vi "Dynamic_Control_Demo.vi"() -> ()   [LabVIEW 2012]
uses:
  <vilib>/Simulation/Scripting/Companion Diagram/SimConfigNode/SimParams.ctl
  <vilib>/Simulation/Scripting/Companion Diagram/SimConfigNode/_simSolvers.ctl
  <vilib>/Simulation/Implementation/Shared/SIMSCR Execution Mode.ctl
  <vilib>/Simulation/Param Hierarchy/Typedefs/SIMPH Param Control Actions.ctl
  <vilib>/Simulation/Implementation/Shared/NILVSim_ParamChanged.vi
  <vilib>/Simulation/DataSources/Implementation/NILVSim Step.llb/SIM Step (scalar).vi
  <vilib>/Simulation/SignalArithmetic/Implementation/NILVSim Gain.llb/SIM Gain (scalar).vi
  <vilib>/Simulation/Utility/Implementation/SIM Halt.vi
  <vilib>/Simulation/DiscreteLinear/Implementation/NILVSim Discrete State Space Buffered.llb/SIM Discrete State Space Distributor (SISO CD).vi
  <vilib>/Simulation/SignalArithmetic/Implementation/NILVSim Gain.llb/SIM Gain (dot product).vi
  <vilib>/Simulation/DiscreteLinear/Implementation/NILVSim Discrete State Space Buffered.llb/SIM Discrete State Space Collector (SISO CD).vi
  <vilib>/Simulation/SignalDisplay/Implementation/NILVSim Time Waveform.llb/SIM Time Waveform (scalar).vi
  <vilib>/Simulation/Implementation/Shared/NILVSim_Manager.vi
  <vilib>/Simulation/Implementation/Shared/NILVSim_FinalizeModel.vi
  <vilib>/Simulation/Implementation/Shared/SIM Unbundle Sim Info.vi
  <vilib>/Utility/error.llb/Clear Errors.vi
  <vilib>/Simulation/Implementation/Shared/NILVSim_GetModelError.vi
  <vilib>/Simulation/Implementation/Shared/SIM Bundle Sim Info.vi
  <vilib>/Simulation/Implementation/Shared/SIMSH Read Queue.vi
  <vilib>/Simulation/Implementation/Shared/NILVSim_Initialize.vi
  <vilib>/Simulation/Utility/Implementation/NILVSim Get Time and IsAcceptedStep.vi
  <vilib>/Simulation/Scripting/Companion Diagram/SimConfigNode/SimDog.xnode
  <vilib>/Simulation/Implementation/XNodeFramework/SimXNode/SimX.xnode
  <vilib>/addons/Control Design/_Model Construction/Model Typedefs.llb/CD General Elements.ctl
  <vilib>/addons/Control Design/_Model Construction/NI_LinSys_Model Typedefs.lvlib
  <vilib>/addons/Control Design/_Model Construction/Model Typedefs.llb/CD State Space Model (MIMO).ctl
  <vilib>/Simulation/DiscreteLinear/Implementation/NILVSim Discrete State Space Buffered.llb/SIM Discrete State Space Buffered (SISO CD).vi
  <vilib>/Simulation/Implementation/Shared/NI_SIM_Implementation.lvlib
panel:
  in  "Halt?":bool
  out "Waveform Plot":waveform(dbl)(graph)={"t0"=timestamp(19414.600000000002 s since 1904-01-01), "dt"=1.0, "Y"=[0.0]}
  out "state x(k+1)":dbl[](array[numeric])
  out "state x(k)":dbl[](array[numeric])
  out "Output y(k)":dbl
  in  "Error IN":dbl(slide) scale=-90.0..90.0
  out "Controllability Matrix":dbl[][](array[numeric])=[[0.0029424877498334255, 0.008616646869548867, 0.014016016852462686, 0.019193532183387766], [0.05829906495647488, 0.05527735475623796, 0.052797981566245, 0.05083784073300338], [0.000983525405599516, 0.0029123179012991098, 0.004844756877997715, 0.006861898357198368], [0.019540617662783182, 0.019171356382024756, 0.019611979984952656, 0.02086921364939449]] format="%.2f"
  out "Feedback Gain (K)":dbl[](array[numeric])=[-63312112.22140336, 6720868.965421855, 193328496.30508494, -20246021.6652911]
  out "Discrete Model Out":picture
  out "Waveform Chart":dbl(graph)
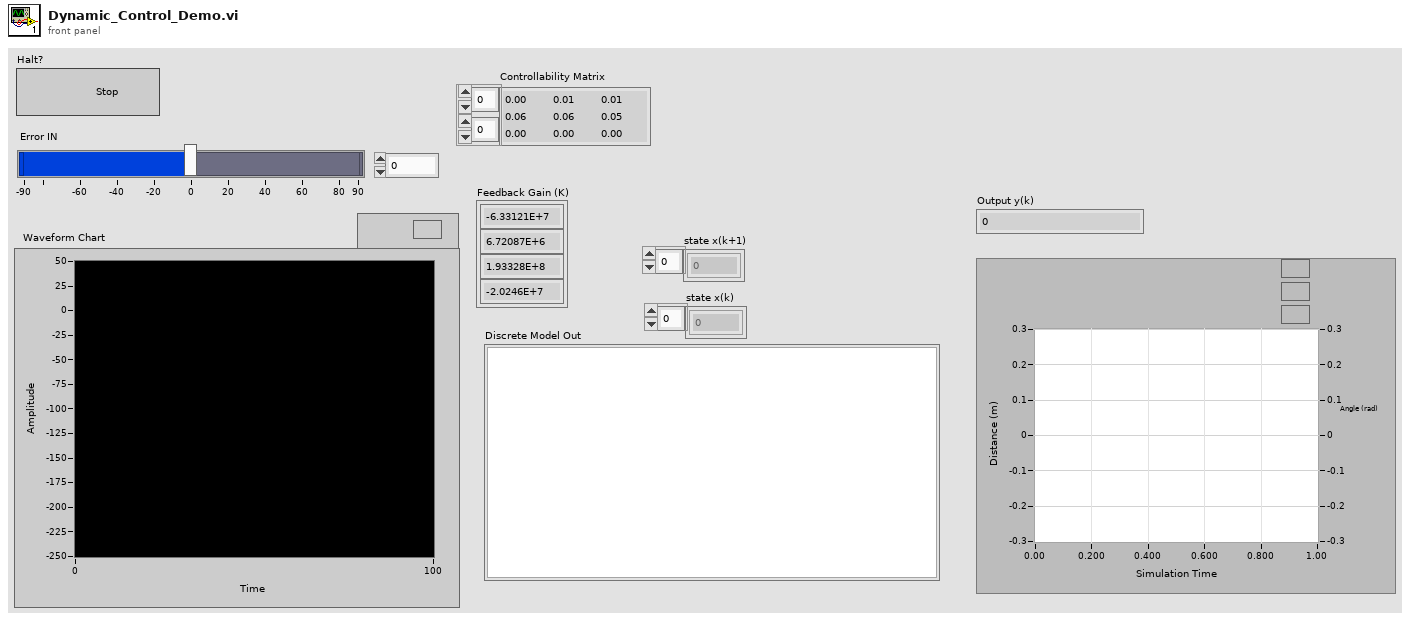
[diagram p1: front panel]
types:
  T1 = typedef "NI_LinSys_Model Typedefs.lvlib/CD State Space Model (MIMO).ctl" = cluster{"properties":T2, "A":dbl[][], "B":dbl[][], "C":dbl[][], "D":dbl[][], "StateNames":string[], "Transport Delay":dbl[][]}
  T2 = typedef "NI_LinSys_Model Typedefs.lvlib/CD General Elements.ctl" = cluster{"Model name":string, "Input names":string[], "Output names":string[], "Input Delays":dbl[], "Output Delays":dbl[], "Sampling Time":dbl, "Notes":string}
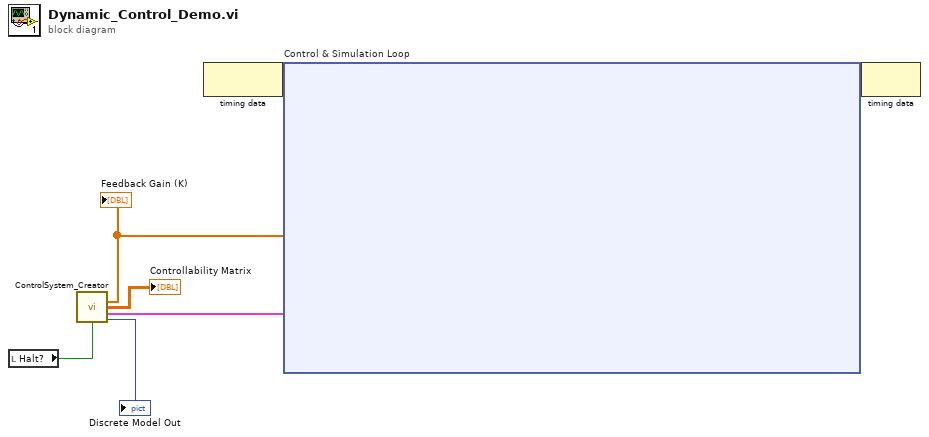
[diagram p0: block diagram]
diagram:
  n1 = local read "Halt?"() -> (w1:bool)
  n2 = call "ControlSystem_Creator.vi"("Stop Button"=w1) -> ("Feedback Gain (K)"=w2:dbl[], "Controllability Matrix"=→"Controllability Matrix":dbl[][], "Discrete State-Space Model"=w5:T1, "Discrete Model Out"=→"Discrete Model Out":picture)  [unwired: 8 in, 3 out]
  "Feedback Gain (K)" <- w2
  n3 = node-c288() -> (w7:variant)  [unwired: 1 in]
  n4 = node-c254 "Control & Simulation Loop"(w7, w5, w2) -> (w6:variant)
  n5 = node-c288(w6) -> ()  [unwired: 1 out]
